vi "Query Multi Eval Meas List TERR Limit Check Results.vi"(8 "error in (no error)":errorcluster, 9 "Result Type (Current)":i32(ring) items=["Current", "Average", "Extreme"], 10 "Instance (1)":T1=1, 11 "VISA resource name":refnum<visa-resource-name>) -> (0 "error out":errorcluster, 1 "Limit Check Results":i32[](array[numeric]), 2 "Reliability":i32, 3 "VISA resource name out":refnum<visa-resource-name>)   [LabVIEW 2020, in "Rohde&Schwarz CMWXP NR FR1 Measurement.lvlib"]
doc: "Return transmit time error limit check results for all measured list mode segments.\n\nAttributes:\nRSCMWXPNRFR1M_ATTR_QUERY_MULTI_EVAL_MEAS_LIST_TERR_CURRENT_LIMIT_CHECK_RESULTS\nRSCMWXPNRFR1M_ATTR_QUERY_MULTI_EVAL_MEAS_LIST_TERR_AVERAGE_LIMIT_CHECK_RESULTS\nRSCMWXPNRFR1M_ATTR_QUERY_MULTI_EVAL_MEAS_LIST_TERR_EXTREME_LIMIT_CHECK_RESULTS\n\nRemote-control commands:\nCALCulate:NRSub:MEAS<i>:MEValuation:LIST:MODulation:TERRor:CURRent?\nCALCulate:NRSub:MEAS<i>:MEValuation:LIST:MODulation:TERRor:AVERage?\nCALCulate:NRSub:MEAS<i>:MEValuation:LIST:MODulation:TERRor:EXTReme?"
uses:
  <instrlib>/Rohde&Schwarz CMWXP NR FR1 Measurement/Rohde&Schwarz CMWXP NR FR1 Measurement.lvlib
  <instrlib>/Rohde&Schwarz CMWXP NR FR1 Measurement/Private/_Instance.ctl
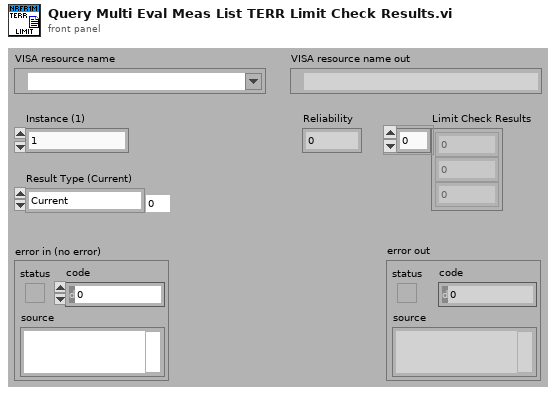
[diagram p1: front panel]
types:
  T1 = typedef "Rohde&Schwarz CMWXP NR FR1 Measurement.lvlib/_Instance.ctl" = i32
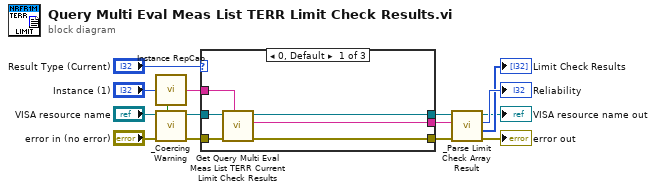
[diagram p0: block diagram]
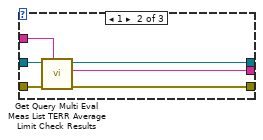
[diagram p2: hidden frame]
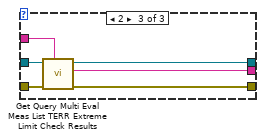
[diagram p3: hidden frame]
diagram:
  n1 = call <instrlib>:"Instance RepCap.vi"("Instance In"="Instance (1)") -> ("In Range?"=w12:bool, "RepCap Identifier Out"=w11:string)  [unwired: 1 in]
  n2 = call <instrlib>:"_Coercing Warning.vi"("In Range?"=w12, "error in (no error)"="error in (no error)", "VISA resource name"="VISA resource name") -> ("error out"=w9:errorcluster, "VISA resource name out"=w10:refnum<visa-resource-name>)  [unwired: 7 in]
  n3 = case shown="0, Default" "Result Type (Current)" {
    tunnel: w11 -> [w21 w27 w33]
    tunnel: w10 -> [w20 w26 w32]
    tunnel: w9 -> [w19 w25 w31]
    tunnel: [w18 w24 w30] -> w5
    tunnel: [w17 w23 w29] -> w6
    tunnel: [w16 w22 w28] -> w7
    frame 0, Default {
      n4 = call "Get Query Multi Eval Meas List TERR Current Limit Check Results"("Repeated Capabilities"=w21, "error in (no error)"=w19, "instrument handle"=w20) -> ("error out"=w16:errorcluster, "Query Multi Eval Meas List TERR Current Limit Check Results"=w17:string, "instrument handle out"=w18:refnum<visa-resource-name>)  [unwired: 6 in]
    }
    frame 1 {
      n5 = call "Get Query Multi Eval Meas List TERR Average Limit Check Results"("Repeated Capabilities"=w27, "error in (no error)"=w25, "instrument handle"=w26) -> ("error out"=w22:errorcluster, "Query Multi Eval Meas List TERR Average Limit Check Results"=w23:string, "instrument handle out"=w24:refnum<visa-resource-name>)  [unwired: 6 in]
    }
    frame 2 {
      n6 = call "Get Query Multi Eval Meas List TERR Extreme Limit Check Results"("Repeated Capabilities"=w33, "error in (no error)"=w31, "instrument handle"=w32) -> ("error out"=w28:errorcluster, "Query Multi Eval Meas List TERR Extreme Limit Check Results"=w29:string, "instrument handle out"=w30:refnum<visa-resource-name>)  [unwired: 6 in]
    }
  }
  n7 = call <instrlib>:"_Parse Limit Check Array Result.vi"("error in (no error)"=w7, "Input String"=w6, "VISA resource name"=w5) -> ("error out"=→"error out":errorcluster, "Results"=→"Limit Check Results":i32[], "Reliability"=→"Reliability":i32, "VISA resource name out"=→"VISA resource name out":refnum<visa-resource-name>)  [unwired: 3 in, 1 out]
